vi "main_with_data_and_queue.vi"() -> ()   [LabVIEW 2024]
panel:
  out "Numeric":dbl
  in  "stop":bool
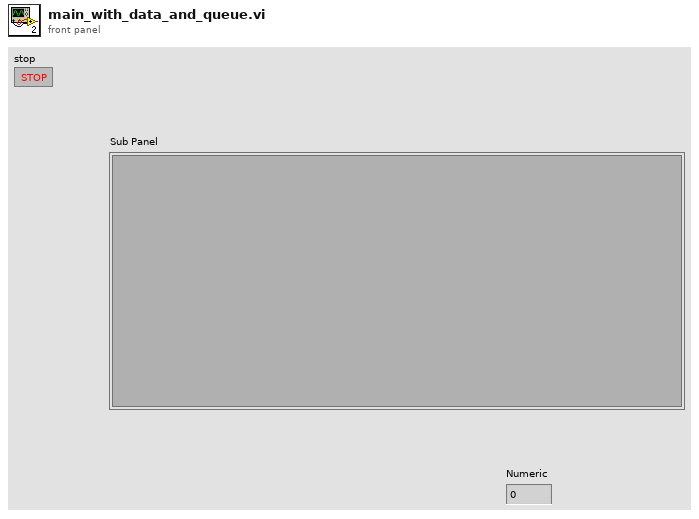
[diagram p1: front panel]
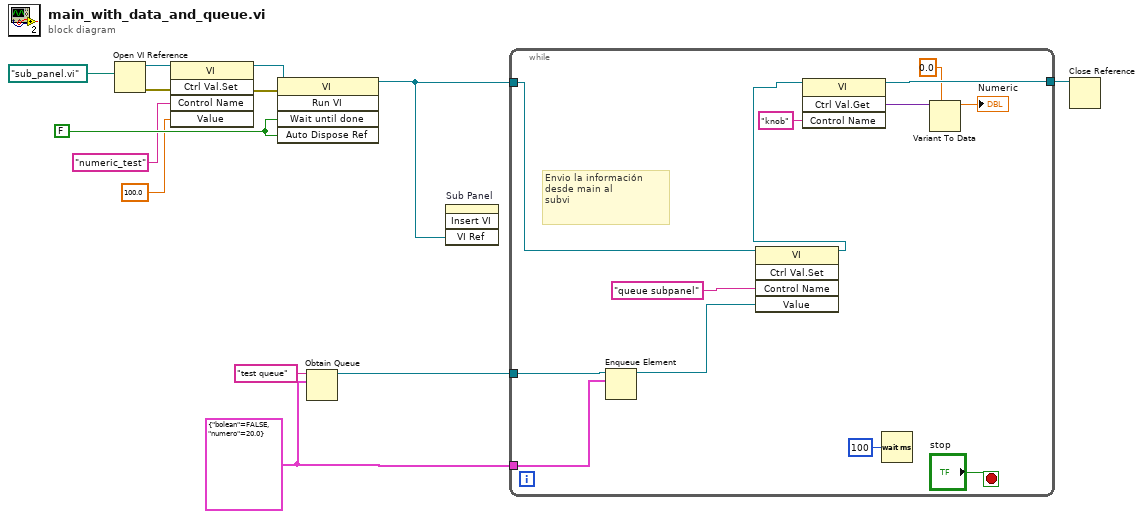
[diagram p0: block diagram]
diagram:
  w1 = cluster{"bolean":bool, "numero":dbl} {"bolean"=FALSE, "numero"=20.0}
  w9 = FALSE ("Wait Until Done")
  n1 = Open VI Reference(vi path=path "sub_panel.vi") -> (vi reference=w11:refnum<vi>, error out=w10:errorcluster)  [unwired: 5 in]
  n2 = invoke class="VI" method="Ctrl Val.Set"(reference=w11, "Control Name"="numeric_test", "Value"=100.0) -> (reference out=w4:refnum<vi>)  [unwired: 2 in, 4 out]
  n3 = invoke class="VI" method="Run VI"(reference=w4, error in=w10, "Wait until done"=w9, "Auto Dispose Ref"=w9) -> (reference out=w8:refnum<vi>)  [unwired: 1 in, 4 out]
  n4 = Obtain Queue(name (unnamed)="test queue", element data type=w1) -> (queue out=w3:refnum<queue>)  [unwired: 3 in, 2 out]
  n5 = invoke on="Sub Panel" class="SubPnl" method="Insert VI"("VI Ref"=w8) -> ()  [unwired: 3 in, 4 out]
  n6 = while {
    tunnel: w8 -> [w13]
    tunnel: [w23] -> w7
    tunnel: w3 -> [w18]
    tunnel: w1 -> [w17]
    stop <- "stop" stop-if-true
    # "Envio la información desde main al \nsubvi"
    n7 = Enqueue Element(queue=w18, element=w17) -> (queue out=w16:refnum<queue>)  [unwired: 2 in, 2 out]
    n8 = invoke class="VI" method="Ctrl Val.Set"(reference=w13, "Control Name"="queue subpanel", "Value"=w16) -> (reference out=w14:refnum<vi>)  [unwired: 2 in, 4 out]
    n9 = invoke class="VI" method="Ctrl Val.Get"(reference=w14, "Control Name"="knob") -> (reference out=w23:refnum<vi>, "Get Control Value Variant"=w21:variant)  [unwired: 2 in, 2 out]
    n10 = Wait (ms)(milliseconds to wait=u32 100) -> ()  [unwired: 1 out]
    n11 = Variant To Data(type=0.0, Variant=w21) -> (data=→"Numeric":dbl)  [unwired: 1 in, 1 out]
  }
  n12 = Close Reference(reference=w7) -> ()  [unwired: 1 in, 1 out]
